vi "S2DS Initialize array inst (SubVI).vi"(8 "error in (no error)":errorcluster, 11 "Instrument parameters in":T1) -> (0 "error out":errorcluster, 3 "Instrument parameters out 2":T1)   [LabVIEW 2016]
uses:
  TYPE DEFS/S2DS_Instrument parameters.ctl
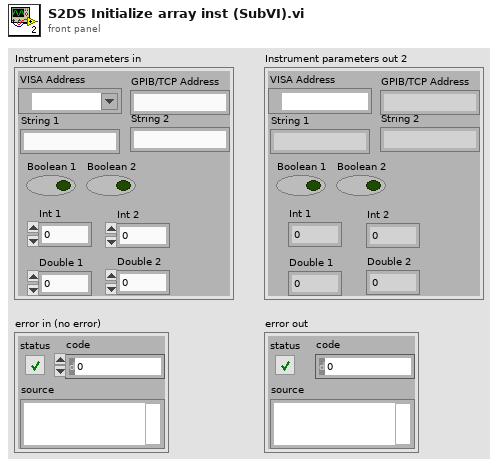
[diagram p1: front panel]
types:
  T1 = typedef "S2DS_Instrument parameters.ctl" = cluster{"VISA Address":refnum<visa-resource-name>, "GPIB/TCP Address":string, "String 1":string, "String 2":string, "Boolean 1":bool, "Boolean 2":bool, "Int 1":i32, "Int 2":i32, "Double 1":dbl, "Double 2":dbl}
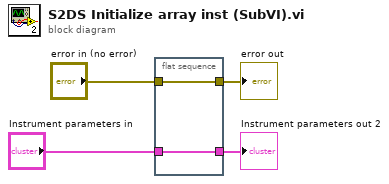
[diagram p0: block diagram]
diagram:
  n1 = flat-sequence {
    tunnel: [w6] -> w2
    tunnel: "error in (no error)" -> [w6]
    tunnel: [w5] -> w4
    tunnel: "Instrument parameters in" -> [w5]
    frame #0 {
    }
  }
  "Instrument parameters out 2" <- w4
  "error out" <- w2
